vi "Database_Status.vi"(8 "error in (no error)":errorcluster) -> (0 "error out":errorcluster, 3 "Test Database":bool)   [LabVIEW 2012]
uses:
  <vilib>/Utility/error.llb/DialogType.ctl
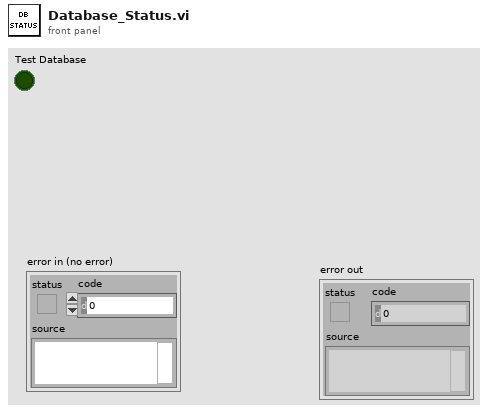
[diagram p1: front panel]
types:
  T1 = typedef "DialogType.ctl" = u16
  T2 = typedef "NI_Database_API.lvlib/Conn ObjectReference.ctl" = refnum<k1>
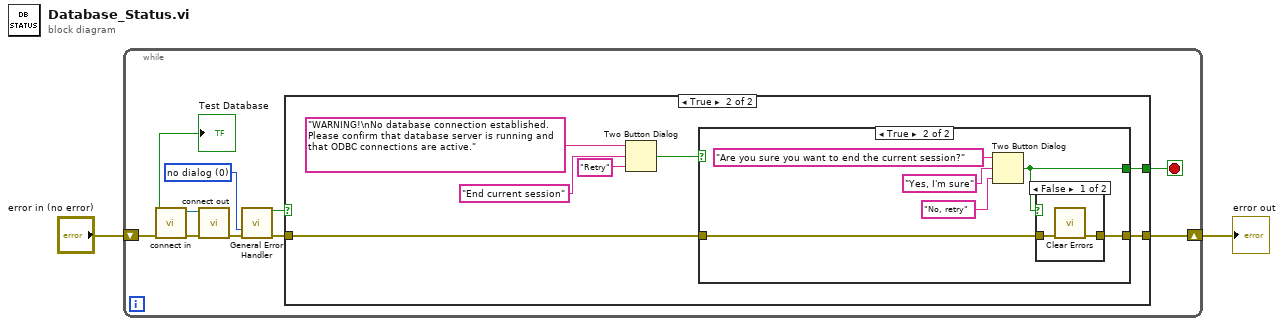
[diagram p0: block diagram]
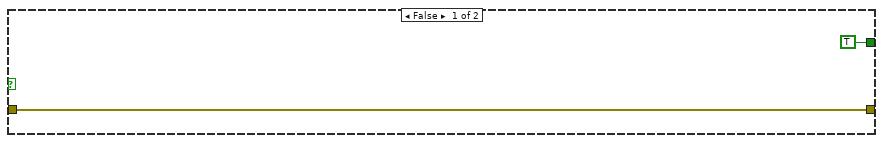
[diagram p2: hidden frame]
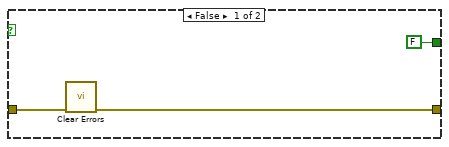
[diagram p3: hidden frame]
diagram:
  n1 = while {
    shift-right: [w3] -> w2
    shift-left: "error in (no error)" -> [w4]
    stop <- w12 stop-if-true
    w6 = T1 0 items=["no dialog", "OK message", "continue or stop message", "OK message + warnings", "continue/stop + warnings"] ("type of dialog (OK msg:1)")
    n2 = call "connect in.vi"("error in (no error)"=w4) -> ("error out"=w10:errorcluster, "Database Connection"=w11:T2, "Test Server"=→"Test Database":bool)  [unwired: 6 in]
    n3 = call "connect out.vi"("error in (no error)"=w10, "connection reference"=w11) -> ("error out"=w9:errorcluster)  [unwired: 9 in]
    n4 = call <vilib>:"General Error Handler.vi"("type of dialog (OK msg:1)"=w6, "error in (no error)"=w9) -> ("error?"=w7:bool, "error out"=w8:errorcluster)  [unwired: 9 in, 3 out]
    n5 = case shown="True" w7 {
      tunnel: [TRUE w17] -> w12
      tunnel: w8 -> [w13 w16]
      tunnel: [w13 w15] -> w3
      frame False {
      }
      frame True {
        n6 = Two Button Dialog(message="WARNING!\nNo database connection established. Please confirm that database server is running and that ODBC connections are active.", 1:"Retry" ("F button name (\"Cancel\")"), 2:"End current session" ("T button name (\"OK\")")) -> (T button?=w18:bool)
        n7 = case shown="True" w18 {
          tunnel: [FALSE w27] -> w17
          tunnel: w16 -> [w23 w26]
          tunnel: [w22 w25] -> w15
          frame False {
            n8 = call <vilib>:"Clear Errors.vi"("error in (no error)"=w23) -> ("error out"=w22:errorcluster)  [unwired: 6 in]
          }
          frame True {
            n9 = Two Button Dialog(message="Are you sure you want to end the current session?", 1:"No, retry" ("F button name (\"Cancel\")"), 2:"Yes, I'm sure" ("T button name (\"OK\")")) -> (T button?=w27:bool)
            n10 = case shown="False" w27 {
              tunnel: w26 -> [w32 w33]
              tunnel: [w31 w33] -> w25
              frame False {
                n11 = call <vilib>:"Clear Errors.vi"("error in (no error)"=w32) -> ("error out"=w31:errorcluster)  [unwired: 6 in]
              }
              frame True {
              }
            }
          }
        }
      }
    }
  }
  "error out" <- w2
